vi "NetworkTables Server.vi"() -> ()   [LabVIEW 2014]
uses:
  <vilib>/Rock Robotics/Network Tables/SD Read Number.vi
panel:
  out "Compared Data":T1(array[cluster])
  in  "Compare":bool
  out "Polar Plot":picture
  in  "Display Scan 2":dbl
  out "Saved Scan 2":picture
  in  "Flagged":T2={"maximum"=500.0, "minimum"=0.0, "clip to min"=FALSE, "log?(F)"=FALSE, "grid color"=6710886, "plot color"=14239, "fmt and prec"={"format"=enum."Decimal", "precision"=0}, "visible section"=8}
  in  "Display Scan":dbl
  in  "Save Scan As":dbl
  out "Saved Data":cluster{"magnitude":dbl, "phase":dbl}[][](array[cluster])
  in  "Live":T2={"maximum"=500.0, "minimum"=0.0, "clip to min"=FALSE, "log?(F)"=FALSE, "grid color"=6710886, "plot color"=16711680, "fmt and prec"={"format"=enum."Decimal", "precision"=0}, "visible section"=8}
  out "Saved Scan":picture
  in  "Saved":T2={"maximum"=500.0, "minimum"=0.0, "clip to min"=FALSE, "log?(F)"=FALSE, "grid color"=6710886, "plot color"=16711680, "fmt and prec"={"format"=enum."Decimal", "precision"=0}, "visible section"=8}
  in  "Take Scan":bool
  out "LIDAR Data":cluster{"magnitude":dbl, "phase":dbl}[](array[cluster])
  out "Live Scan":picture
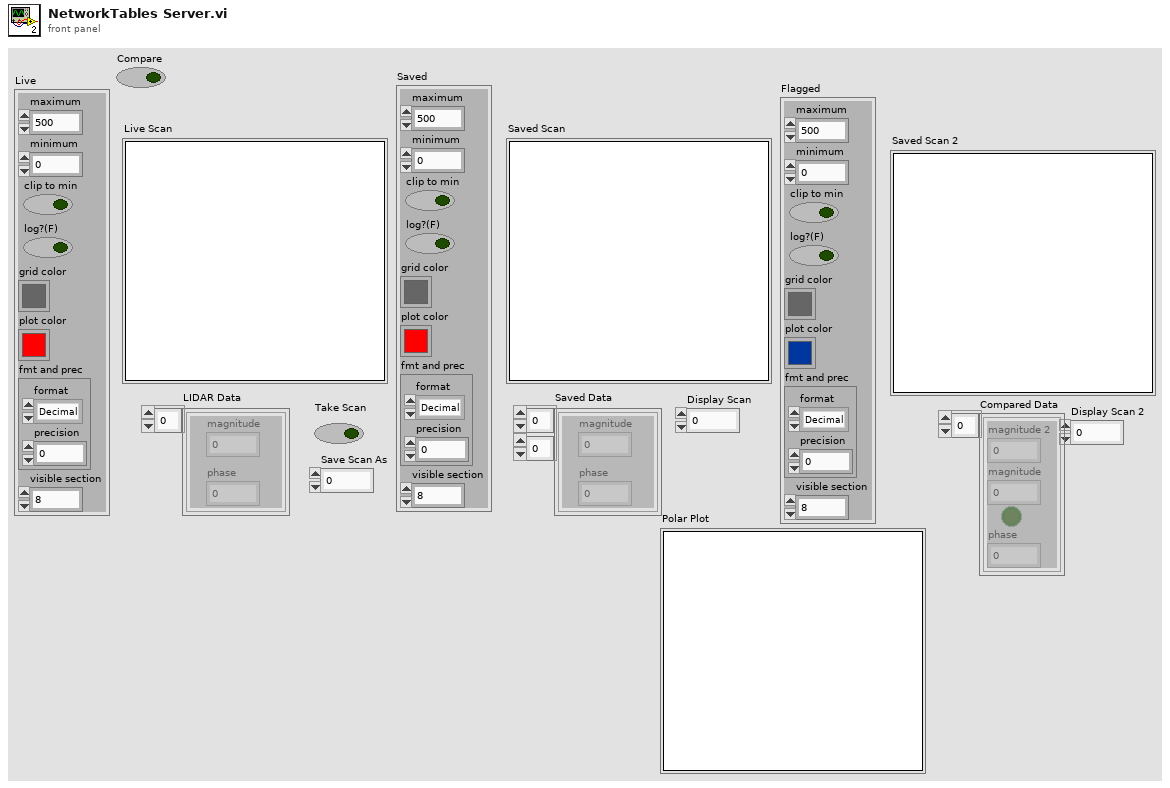
[diagram p1: front panel]
types:
  T1 = cluster{"magnitude 2":dbl, "magnitude":dbl, "flagged":bool, "phase":dbl}[]
  T2 = cluster{"maximum":dbl, "minimum":dbl, "clip to min":bool, "log?(F)":bool, "grid color":u32, "plot color":u32, "fmt and prec":cluster{"format":enum8{"Decimal", "Scientific", "Engineering", "Binary", "Octal", "Hex"}, "precision":u8}, "visible section":u16}
  T3 = cluster{"[0]":i32, "[1]":i32, "[2]":i32, "[3]":i32, "[4]":i32, "[5]":i32, "[6]":i32, "[7]":i32, "[8]":i32}
  T4 = cluster{"magnitude":dbl, "magnitude":dbl, bool, "phase":dbl}
  T5 = typedef "LVBoundsTypeDef.ctl" = cluster{"Width":u32, "Height":u32}
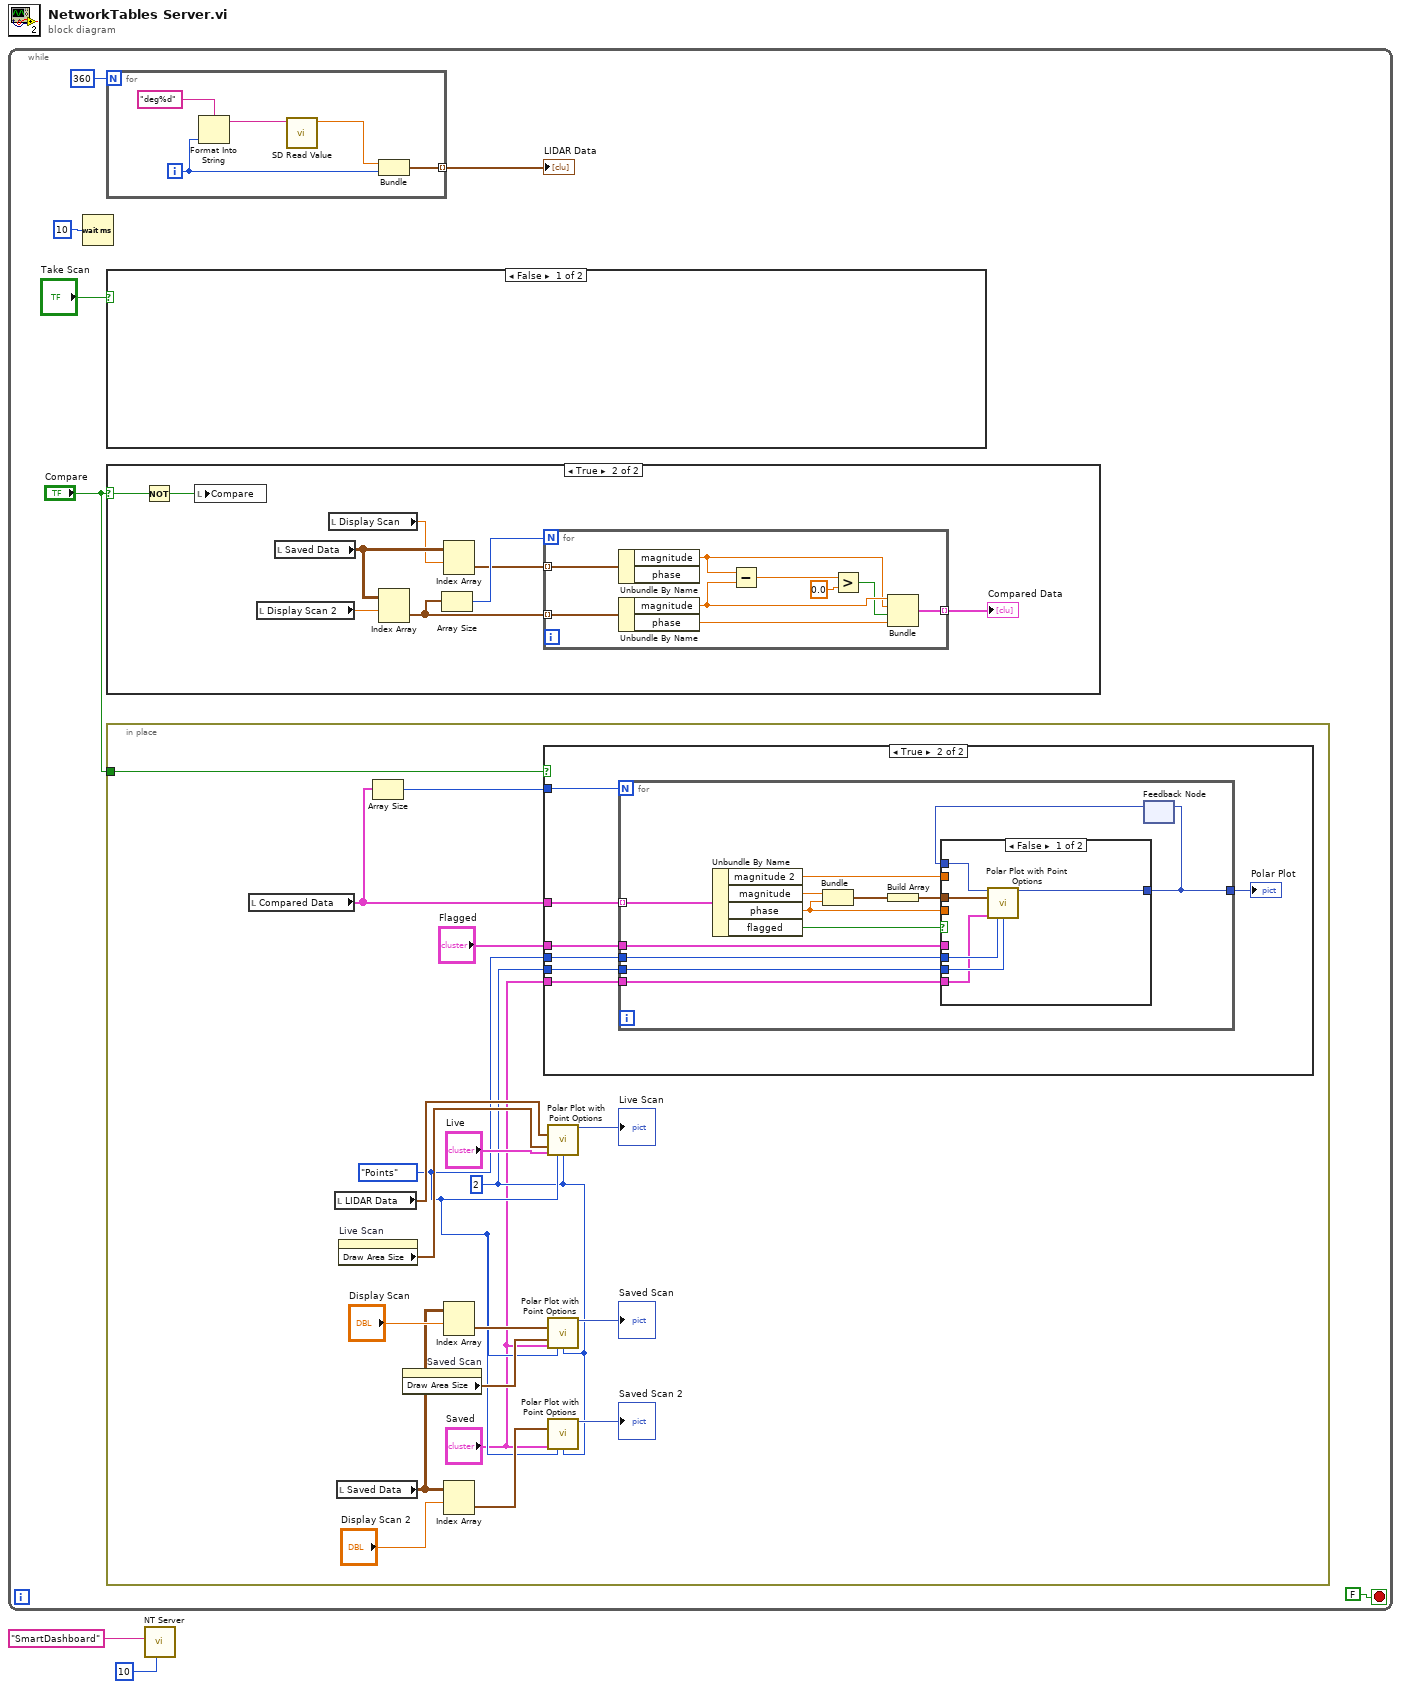
[diagram p0: block diagram]
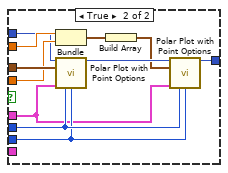
[diagram p4: hidden frame]
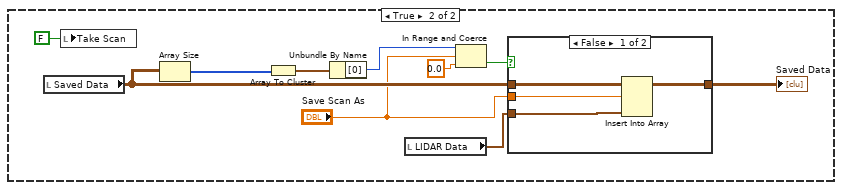
[diagram p5: hidden frame]
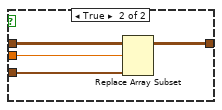
[diagram p6: hidden frame]
diagram:
  n1 = while {
    stop <- FALSE stop-if-true
    n2 = Wait (ms)(milliseconds to wait=u32 10) -> ()  [unwired: 1 out]
    n3 = for {
      N: 360 -> [_]
      tunnel: [w101] -> w5 mode=indexing
      i -> [w102]
      n4 = Format Into String(format string="deg%d", w102) -> (resulting string=w104:string)  [unwired: 2 in, 1 out]
      n5 = call-poly <vilib>:"SD Read Value.vi"("Name"=w104) -> ("Numeric"=w103:dbl)  [unwired: 8 in, 2 out]
      n6 = Bundle("Numeric"=w103, w102) -> (w101:cluster{"Numeric":dbl, i32})  [unwired: 1 in]
    }
    "LIDAR Data" <- w5
    n7 = case shown="False" "Take Scan" {
      frame False {
      }
      frame True {
        n8 = local read "Saved Data"() -> (w85:cluster{"magnitude":dbl, "phase":dbl}[][])
        n9 = local write "Take Scan"(FALSE) -> ()
        n10 = Array Size(array=w85) -> (size(s)=w91:i32[])
        n11 = Array To Cluster(array=w91) -> (cluster=w90:T3)
        n12 = Unbundle By Name(w90) -> ("[0]"=w89:i32)
        n13 = local read "LIDAR Data"() -> (w86:cluster{"magnitude":dbl, "phase":dbl}[])
        n14 = In Range and Coerce(upper limit=w89, x="Save Scan As", lower limit=0.0) -> (In Range?=w88:bool)  [unwired: 1 out]
        n15 = case shown="False" w88 {
          tunnel: w86 -> [w94 w100]
          tunnel: w85 -> [w95 w99]
          tunnel: "Save Scan As" -> [w96 w98]
          tunnel: [w93 w97] -> w83
          frame False {
            n16 = Insert Into Array(array=w95, index (row)=w96, new element=w94) -> (w93:cluster{"magnitude":dbl, "phase":dbl}[][])  [unwired: 1 in]
          }
          frame True {
            n17 = Replace Array Subset(array=w99, new element=w100, index (row)=w98) -> (w97:cluster{"magnitude":dbl, "phase":dbl}[][])  [unwired: 1 in]
          }
        }
        "Saved Data" <- w83
      }
    }
    n18 = case shown="True" "Compare" {
      selector: "Compare" -> [_ w10]
      frame False {
      }
      frame True {
        n19 = Not(x=w10) -> (.not. x?=w9:bool)
        n20 = local write "Compare"(w9) -> ()
        n21 = local read "Display Scan 2"() -> (w15:dbl)
        n22 = local read "Saved Data"() -> (w17:cluster{"magnitude":dbl, "phase":dbl}[][])
        n23 = local read "Display Scan"() -> (w16:dbl)
        n24 = Index Array(array=w17, index (row)=w15) -> (element=w14:cluster{"magnitude":dbl, "phase":dbl}[])  [unwired: 1 in]
        n25 = Array Size(array=w14) -> (size(s)=w13:i32)
        n26 = Index Array(array=w17, index (row)=w16) -> (element=w12:cluster{"magnitude":dbl, "phase":dbl}[])  [unwired: 1 in]
        n27 = for {
          N: w13 -> [_]
          tunnel: w14 -> [w26] mode=indexing
          tunnel: w12 -> [w25] mode=indexing
          tunnel: [w19] -> w11 mode=indexing
          n28 = Unbundle By Name(w25) -> ("magnitude"=w20:dbl)  [unwired: 1 out]
          n29 = Unbundle By Name(w26) -> ("magnitude"=w22:dbl, "phase"=w21:dbl)
          n30 = Subtract(x=w20, y=w22) -> (x-y=w24:dbl)
          n31 = Greater?(x=w24, y=0.0) -> (0:w18:bool)
          n32 = Bundle("magnitude"=w22, "magnitude"=w20, w18, "phase"=w21) -> (w19:T4)  [unwired: 1 in]
        }
        "Compared Data" <- w11
      }
    }
    n33 = in-place {
      in-place-border: "Compare" -> [w27]
      w30 = 2
      w31 = enum16{"Lines", "Points"}."Points" ("Lines/Points")
      n34 = local read "Compared Data"() -> (w32:T1)
      n35 = local read "LIDAR Data"() -> (w43:cluster{"magnitude":dbl, "phase":dbl}[])
      n36 = local read "Saved Data"() -> (w36:cluster{"magnitude":dbl, "phase":dbl}[][])
      n37 = property on="Live Scan" class="Pict"() -> ("Draw Area Size"=w44:T5)  [unwired: 2 in, 2 out]
      n38 = Array Size(array=w32) -> (size(s)=w33:i32)
      n39 = property on="Saved Scan" class="Pict"() -> ("Draw Area Size"=w42:T5)  [unwired: 2 in, 2 out]
      n40 = Index Array(array=w36, index (row)="Display Scan") -> (element=w38:cluster{"magnitude":dbl, "phase":dbl}[])  [unwired: 1 in]
      n41 = Index Array(array=w36, index (row)="Display Scan 2") -> (element=w35:cluster{"magnitude":dbl, "phase":dbl}[])  [unwired: 1 in]
      n42 = case shown="True" w27 {
        tunnel: w33 -> [_ w52]
        tunnel: w32 -> [_ w51]
        tunnel: w31 -> [_ w50]
        tunnel: w30 -> [_ w49]
        tunnel: "Flagged" -> [_ w48]
        tunnel: "Saved" -> [_ w47]
        frame False {
        }
        frame True {
          n43 = for {
            N: w52 -> [_]
            tunnel: w51 -> [w65] mode=indexing
            tunnel: w50 -> [w59]
            tunnel: w49 -> [w58]
            tunnel: w48 -> [w57]
            tunnel: w47 -> [w56]
            tunnel: [w54] -> w46
            n44 = Unbundle By Name(w65) -> ("magnitude 2"=w61:dbl, "magnitude"=w64:dbl, "phase"=w60:dbl, "flagged"=w53:bool)
            n45 = Bundle("magnitude"=w64, "phase"=w60) -> (w62:cluster{"magnitude":dbl, "phase":dbl})  [unwired: 1 in]
            n46 = Build Array(w62) -> (w63:cluster{"magnitude":dbl, "phase":dbl}[])
            n47 = feedback #1() -> (w55:picture)  [unwired: 1 in]
            n48 = case shown="False" w53 {
              tunnel: w63 -> [w71 w82]
              tunnel: w61 -> [_ w81]
              tunnel: w60 -> [_ w80]
              tunnel: w59 -> [w69 w76]
              tunnel: w58 -> [w70 w75]
              tunnel: w57 -> [_ w74]
              tunnel: w56 -> [w68 _]
              tunnel: [w67 w73] -> w54
              tunnel: w55 -> [w66 w72]
              frame False {
                n49 = call <vilib>:"Polar Plot with Point Options.vi"("picture"=w66, "data array [mag, phase (deg)]"=w71, "polar attributes"=w68, "Lines/Points"=w69, "Size"=w70) -> ("new picture"=w67:picture)  [unwired: 10 in]
              }
              frame True {
                n50 = Bundle("magnitude 2"=w81, "phase"=w80) -> (w79:cluster{"magnitude 2":dbl, "phase":dbl})  [unwired: 1 in]
                n51 = call <vilib>:"Polar Plot with Point Options.vi"("picture"=w72, "data array [mag, phase (deg)]"=w82, "polar attributes"=w74, "Lines/Points"=w76, "Size"=w75) -> ("new picture"=w78:picture)  [unwired: 10 in]
                n52 = Build Array(w79) -> (w77:cluster{"magnitude 2":dbl, "phase":dbl}[])
                n53 = call <vilib>:"Polar Plot with Point Options.vi"("picture"=w78, "data array [mag, phase (deg)]"=w77, "polar attributes"=w74, "Lines/Points"=w76, "Size"=w75) -> ("new picture"=w73:picture)  [unwired: 10 in]
              }
            }
            n54 = feedback-in #1(w54) -> ()
          }
          "Polar Plot" <- w46
        }
      }
      n55 = call <vilib>:"Polar Plot with Point Options.vi"("data array [mag, phase (deg)]"=w43, "dimensions (w,h)"=w44, "polar attributes"="Live", "Lines/Points"=w31, "Size"=w30) -> ("new picture"=→"Live Scan":picture)  [unwired: 10 in]
      n56 = call <vilib>:"Polar Plot with Point Options.vi"("data array [mag, phase (deg)]"=w38, "dimensions (w,h)"=w42, "polar attributes"="Saved", "Lines/Points"=w31, "Size"=w30) -> ("new picture"=→"Saved Scan":picture)  [unwired: 10 in]
      n57 = call <vilib>:"Polar Plot with Point Options.vi"("data array [mag, phase (deg)]"=w35, "polar attributes"="Saved", "Lines/Points"=w31, "Size"=w30) -> ("new picture"=→"Saved Scan 2":picture)  [unwired: 11 in]
    }
  }
  n58 = call <vilib>:"NT Server.vi"("Update Time"=10, "Server Name"="SmartDashboard") -> ()  [unwired: 10 in]
